vi "Post-Build Action.vi"(5 "Files Generated by Build":path[](array[path]), 6 "Top Level/Always Included VIs":path[](array[path]), 7 "Destination Path":path, 8 "error in (no error)":errorcluster, 9 "Target Name":string, 10 "Build Specification Name":string, 11 "Project Path":path) -> (0 "error out":errorcluster)   [LabVIEW 2015]
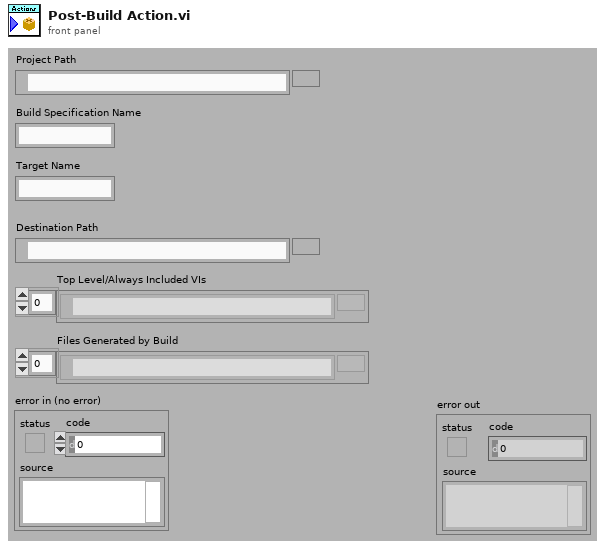
[diagram p1: front panel]
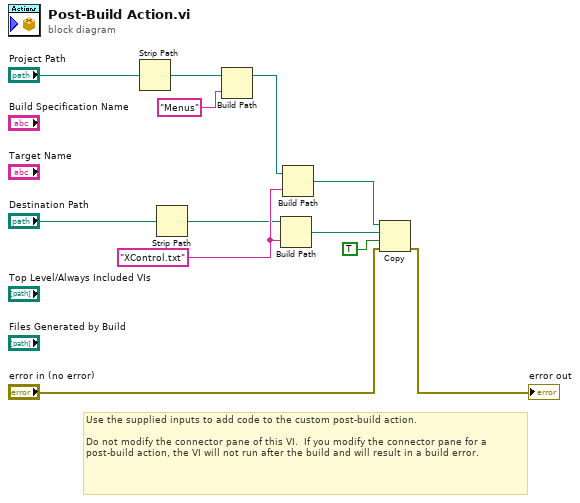
[diagram p0: block diagram]
diagram:
  w7 = "XControl.txt" ("name or relative path")
  # "Use the supplied inputs to add code to the custom post-build action.\n\nDo not modify the connector pane of this VI.  If you modify the connector pane for a post-build action, the VI will not run after the build and will result in a build error."
  n1 = Strip Path(path="Project Path") -> (stripped path=w5:path)  [unwired: 1 out]
  n2 = Strip Path(path="Destination Path") -> (stripped path=w4:path)  [unwired: 1 out]
  n3 = Build Path(base path=w5, name or relative path="Menus") -> (appended path=w2:path)
  n4 = Build Path(base path=w4, name or relative path=w7) -> (appended path=w8:path)
  n5 = Build Path(base path=w2, name or relative path=w7) -> (appended path=w6:path)
  n6 = Copy(8:"error in (no error)", 9:TRUE ("overwrite (F)"), 10:w8, 11:w6) -> (0:→"error out":errorcluster)  [unwired: 1 in, 2 out]
